vi "ATF-Pump-CDT HOLD FGV.vi"(5 "Write/Read":enum16{"Write", "Read"}(ring), 6 "error in (no error)":errorcluster, 8 "HOLD and Abort":T1) -> (0 "error Out":errorcluster, 2 "HOLD and Abort Out":T1)   [LabVIEW 2022 SP3]
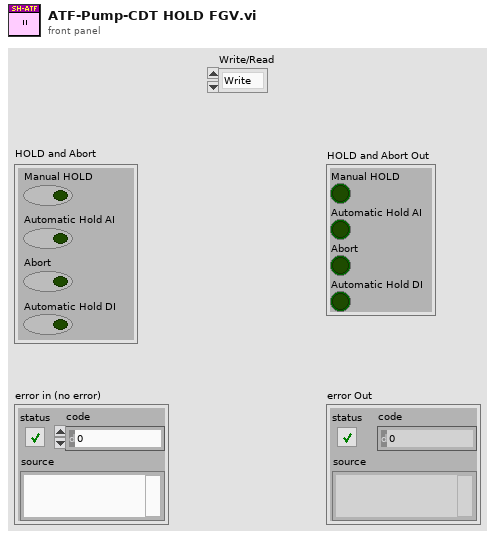
[diagram p1: front panel]
types:
  T1 = cluster{"Manual HOLD":bool, "Automatic Hold AI":bool, "Abort":bool, "Automatic Hold DI":bool}
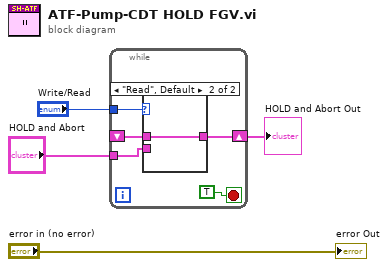
[diagram p0: block diagram]
diagram:
  n1 = while {
    tunnel: "Write/Read" -> [w8]
    shift-right: [w6] -> w1
    shift-left: _ -> [w7]
    tunnel: "HOLD and Abort" -> [w5]
    stop <- TRUE stop-if-true
    n2 = case shown="\"Read\", Default" w8 {
      tunnel: w7 -> [_ w11]
      tunnel: [w10 w11] -> w6
      tunnel: w5 -> [w10 _]
      frame "Write" {
      }
      frame "Read", Default {
      }
    }
  }
  "HOLD and Abort Out" <- w1
  "error Out" <- "error in (no error)"
